vi "Programming1.vi"(7 "DUT1?":bool=TRUE, 8 "error in":errorcluster, 9 "Supply PCB over Programator":bool, 10 "Family":string, 11 "FileName":string) -> (0 "error out":errorcluster, 1 "Programming passed":bool, 2 "standard error":string, 3 "standard output":string)   [LabVIEW 2023]
panel:
  out "return code":i32
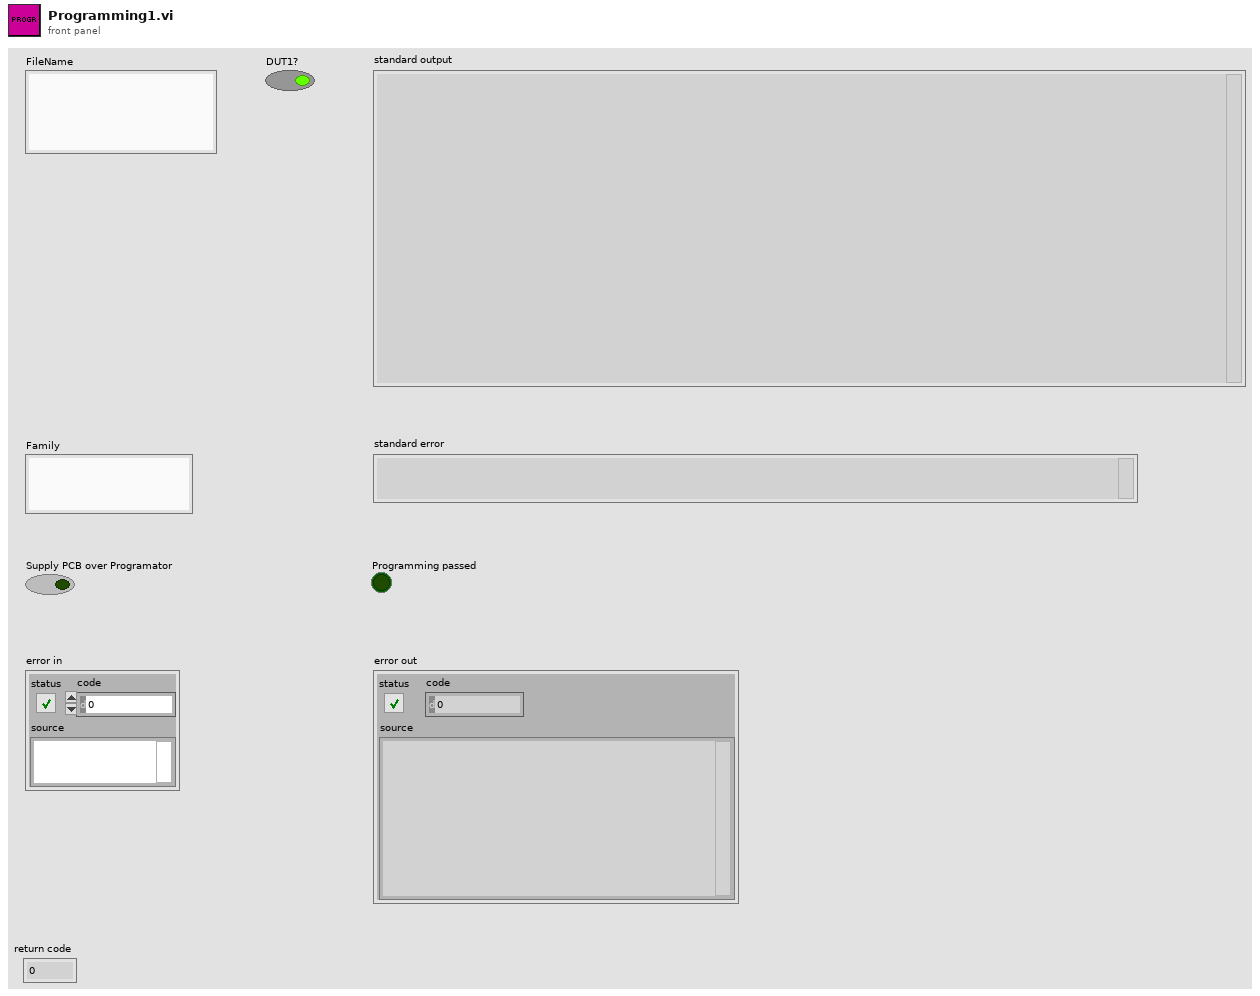
[diagram p1: front panel]
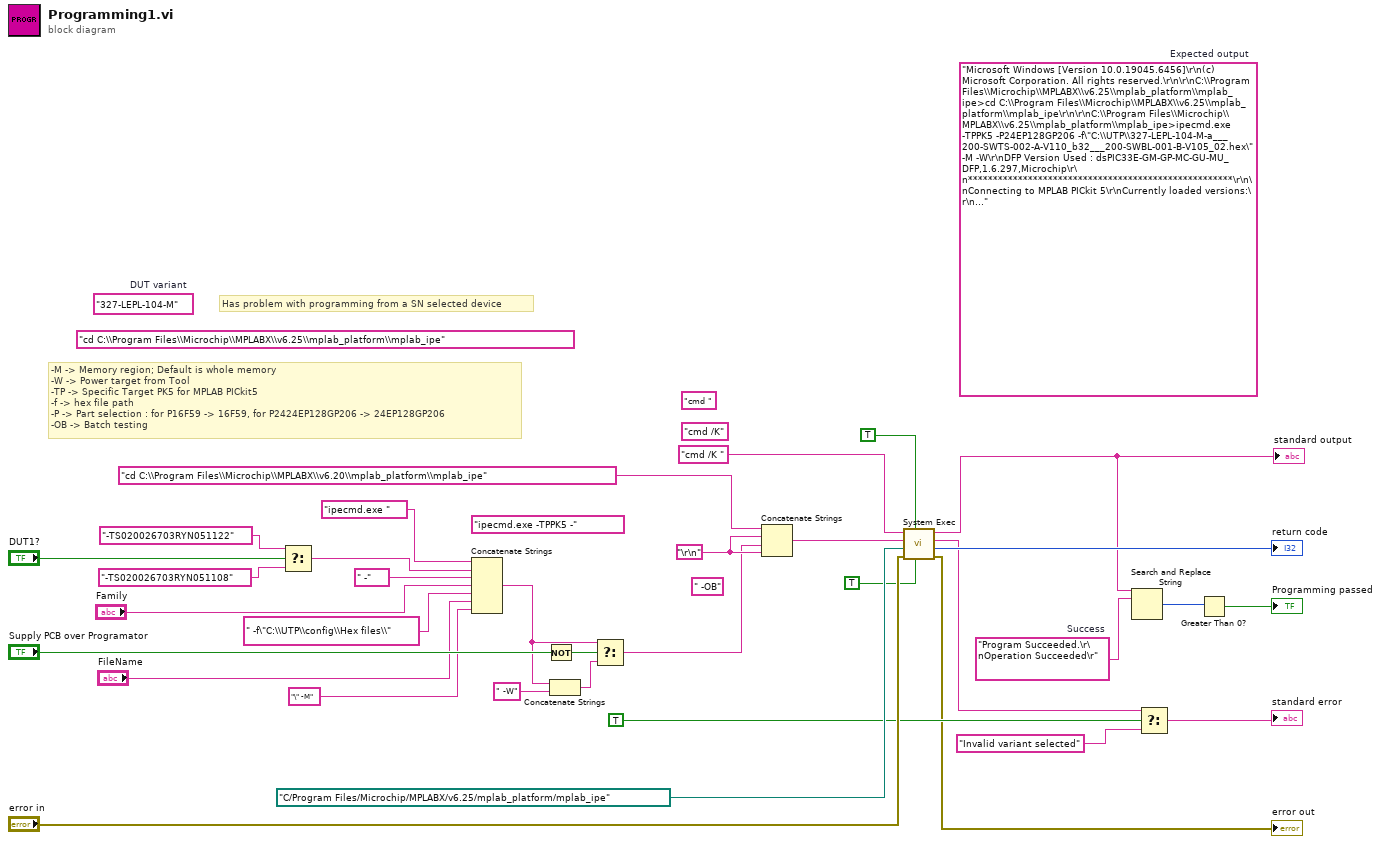
[diagram p0: block diagram]
diagram:
  (unwired) "cmd " ("command line")
  (unwired) "ipecmd.exe -TPPK5 -" ("command line")
  (unwired) "cd C:\\Program Files\\Microchip\\MPLABX\\v6.25\\mplab_platform\\mplab_ipe" ("command line")
  (unwired) "cmd /K" ("command line")
  (unwired) " -OB" ("string")
  w20 = "Program Succeeded.\r\nOperation Succeeded\r"  # Success
  (unwired) "Microsoft Windows [Version 10.0.19045.6456]\r\n(c) Microsoft Corporation. All rights reserved.\r\n\r\nC:\\Program Files\\Microchip\\MPLABX\\v6.25\\mplab_platform\\mplab_ipe>cd C:\\Program Files\\Microchip\\MPLABX\\v6.25\\mplab_platform\\mplab_ipe\r\n\r\nC:\\Program Files\\Microchip\\MPLABX\\v6.25\\mplab_platform\\mplab_ipe>ipecmd.exe -TPPK5 -P24EP128GP206 -f\"C:\\UTP\\327-LEPL-104-M-a___200-SWTS-002-A-V110_b32___200-SWBL-001-B-V105_02.hex\" -M -W\r\nDFP Version Used : dsPIC33E-GM-GP-MC-GU-MU_DFP,1.6.297,Microchip\r\n*****************************************************\r\n\nConnecting to MPLAB PICkit 5\r\nCurrently loaded versions:\r\nApplication version...........02.04.54\r\nBoot version..................00.00.68\r\nPCB version...................3\r\nScript version................00.08.91\r\nScript build number...........0674c1b56b\r\nTool pack version ............2.9.699\r\nBLE version ..................1.44\r\nPICkit 5 is supplying power to the target (3.25 volts).\r\nTarget device PIC24EP128GP206 found.\r\nDevice Revision Id  = 0x4008\r\nDevice Id = 0x1e5b0000\r\n*****************************************************\r\nCalculating memory ranges for operation...\r\nErasing...\r\nThe following memory area(s) will be programmed:\r\nprogram memory: start address = 0x0, end address = 0x7ff\nprogram memory: start address = 0x1000, end address = 0x97ff\nprogram memory: start address = 0x13800, end address = 0x13fff\nprogram memory: start address = 0x14800, end address = 0x157eb\nconfiguration memory\nUser Id Memory\r\nProgramming/Verify complete\r\n Program Report\r\n2026-01-16, 11:57:39\r\nDevice Type:PIC24EP128GP206\r\nProgram Succeeded.\r\nOperation Succeeded\r\n\r\nC:\\Program Files\\Microchip\\MPLABX\\v6.25\\mplab_platform\\mplab_ipe>"  # Expected output
  (unwired) "327-LEPL-104-M"  # DUT variant
  w16 = "\r\n"
  # "Has problem with programming from a SN selected device"
  # "-M -> Memory region; Default is whole memory\n-W -> Power target from Tool\n-TP -> Specific Target PK5 for MPLAB PICkit5\n-f -> hex file path\n-P -> Part selection : for P16F59 -> 16F59, for P2424EP128GP206 -> 24EP128GP206\n-OB -> Batch testing"
  n1 = Select(t="-TS020026703RYN051122" ("command line"), s="DUT1?", f="-TS020026703RYN051108" ("command line")) -> (s? t:f=w2:string)
  n2 = Concatenate Strings("ipecmd.exe " ("command line"), w2, " -" ("command line"), "Family", " -f\"C:\\UTP\\config\\Hex files\\" ("command line"), "FileName", "\" -M" ("string")) -> (w8:string)
  n3 = Not(x="Supply PCB over Programator") -> (.not. x?=w27:bool)
  n4 = Concatenate Strings(w8, " -W" ("string")) -> (w13:string)
  n5 = Select(t=w8, s=w27, f=w13) -> (s? t:f=w15:string)
  n6 = Concatenate Strings("cd C:\\Program Files\\Microchip\\MPLABX\\v6.20\\mplab_platform\\mplab_ipe" ("command line"), w16, w15, w16) -> (w30:string)
  n7 = call <vilib>:"System Exec.vi"("run minimized? (F)"=TRUE, "wait until completion? (T)"=TRUE, "error in (no error)"="error in", "working directory"=path "C:/Program Files/Microchip/MPLABX/v6.25/mplab_platform/mplab_ipe", "standard input"=w30, "command line"="cmd /K ") -> ("error out"=→"error out":errorcluster, "return code"=→"return code":i32, "standard error"=w23:string, "standard output"=w21:string)  [unwired: 2 in]
  "standard output" <- w21
  n8 = Search and Replace String(input string=w21, search string=w20) -> (number of replacements=w19:i32)  [unwired: 6 in, 3 out]
  n9 = Select(t=w23, s=TRUE, f="Invalid variant selected") -> (s? t:f=→"standard error":string)
  n10 = Greater Than 0?(x=w19) -> (x > 0?=→"Programming passed":bool)
